vi "Set Graph Legend Entries.vi"(0 "Graph Reference":refnum<vi>, 1 "Legend Entries":string[](array[string])) -> ()   [LabVIEW 2013]
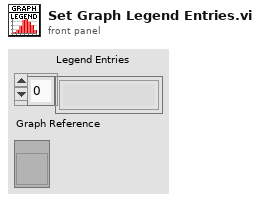
[diagram p1: front panel]
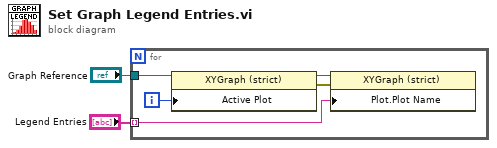
[diagram p0: block diagram]
diagram:
  n1 = for {
    tunnel: "Graph Reference" -> [w7]
    tunnel: "Legend Entries" -> [w3] mode=indexing
    i -> [w6]
    n2 = property class="XYGraph (strict)"(reference=w7, "Active Plot"=w6) -> (reference out=w5:refnum<vi>, error out=w4:errorcluster)  [unwired: 1 in]
    n3 = property class="XYGraph (strict)"(reference=w5, error in=w4, "Plot.Plot Name"=w3) -> ()  [unwired: 2 out]
  }
